vi "Do.vi"(8 "error in":errorcluster, 10 "Actor in":refnum<class "Actor.lvclass">, 11 "Toggle Filter Cycle MSG":refnum<class "Toggle Filter Cycle MSG.lvclass">) -> (0 "error out":errorcluster, 2 "Actor out":refnum<class "Actor.lvclass">)   [LabVIEW 2014, in "Controller.lvlib" / "Toggle Filter Cycle MSG.lvclass"]
doc: "(<B>Filename</B>: Actor Framework.lvlib:Message.lvclass:Do.vi)\n\nDefines what a message does when it is received by an actor. Generally, a message instructs an actor to invoke one of its methods. By default, this method does nothing. A child class must override it to define behavior. Create a child class by using the Actor Framework Message Maker dialog box."
uses:
  Toggle Filter Cycle MSG.lvclass
  <vilib>/ActorFramework/Actor/Actor.lvclass
  Toggle Filter Cycle MSG.lvclass/Toggle Filter Cycle MSG.ctl
  Controller.lvclass
  Controller.lvclass/Controller.ctl
  SuperActor/SuperActor.lvclass/SuperActor.ctl
  reusable/Switch/Switch.lvclass/Switch.ctl
  reusable/Switch/Write Cycle_.vi
  Accessors/Read Switch DVR.vi
  SuperActor/Read Log Session.vi
  SuperActor/Read CVT Session.vi
  <userlib>/_Session Fwk/Session - Root.lvclass
  reusable/Switch/Switch.lvclass
  reusable/Session APIs/Session Log/System Log.lvclass
  reusable/Session APIs/CVT/CVT.lvclass
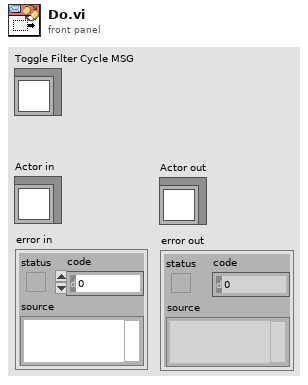
[diagram p1: front panel]
types:
  T1 = typedef "Session - Root.lvclass/Session Handle.ctl" = refnum<data-value>
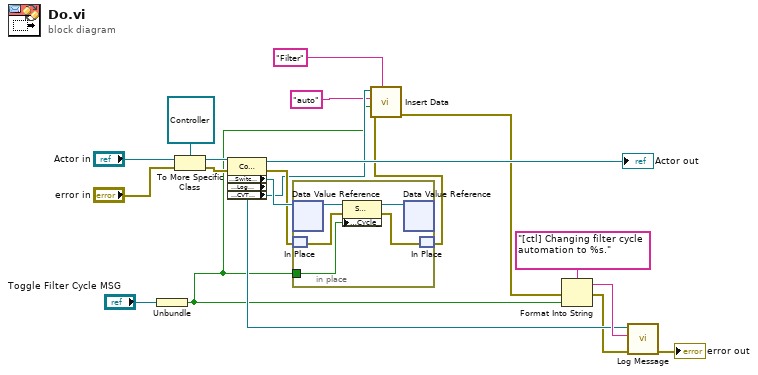
[diagram p0: block diagram]
diagram:
  n1 = Unbundle("Toggle Filter Cycle MSG") -> (w4:bool)
  n2 = To More Specific Class(target class=refnum<class "Controller.lvclass"> refnum ("Controller.lvlib:Controller"), reference="Actor in", error in="error in") -> (specific class reference=w19:refnum<class "Controller.lvclass">, error out=w18:errorcluster)
  n3 = property class="Controller"(reference=w19, error in=w18) -> (reference out=→"Actor out":refnum<class "Controller.lvclass">, error out=w8:errorcluster, "Accessors:Switch DVR"=w16:refnum<data-value>, "Accessors:Log Session"=w10:T1, "Accessors:CVT Session"=w7:T1)
  n4 = in-place {
    in-place-border: w4 -> [w23]
    n5 = in-place-dvr #1(w16) -> (w25:refnum<class "Switch.lvclass">)  [unwired: 1 out]
    n6 = in-place-match #2(w8) -> (w22:errorcluster)
    n7 = property class="Switch"(reference=w25, error in=w22, "Accessors:Cycle_"=w23) -> (reference out=w24:refnum<class "Switch.lvclass">, error out=w21:errorcluster)
    n8 = in-place-dvr #1(w24) -> ()  [unwired: 2 out]
    n9 = in-place-match #2(w21) -> (w3:errorcluster)
  }
  n10 = call "Insert Data.vi"("Group"="Filter", "error in"=w3, "Data"=w4, "tag"="auto", "CVT Session In"=w7) -> ("error out"=w2:errorcluster)  [unwired: 5 in, 1 out]
  n11 = Format Into String(format string="[ctl] Changing filter cycle automation to %s.", error in=w2, w4) -> (resulting string=w11:string, error out=w9:errorcluster)  [unwired: 1 in]
  n12 = call "Log Message.vi"("error in"=w9, "MSG In"=w11, "session in"=w10) -> ("error out"=→"error out":errorcluster)  [unwired: 7 in, 1 out]
